vi "Launcher - gRPC Client.vi"(6 "Worker Alias":string="gRPC Client", 8 "error in":errorcluster, 9 "Initialization Data":T1, 11 "gRPC Client in":refnum<class "gRPC Client.lvclass">) -> (0 "error out":errorcluster)   [LabVIEW 2023]
doc: "This VI launches the Head Worker of a Workers application."
uses:
  Workers/gRPC Client/Initialization Data.ctl
  Workers/gRPC Client/Response Cases.ctl
  <vilib>/gRPC/LabVIEW gRPC Library/Shared/grpcId.ctl
  Workers/gRPC Client/gRPC Client.lvclass
  C:/Program Files (x86)/National Instruments/LabVIEW 2023/vi.lib/addons/_Workers/Library/Classes/Worker/Worker.lvclass
  <vilib>/addons/_Workers/Debugger/Debug Client/Debug Client.lvlib
  <vilib>/gRPC/LabVIEW gRPC Library/grpc-lvsupport-release.lvlib
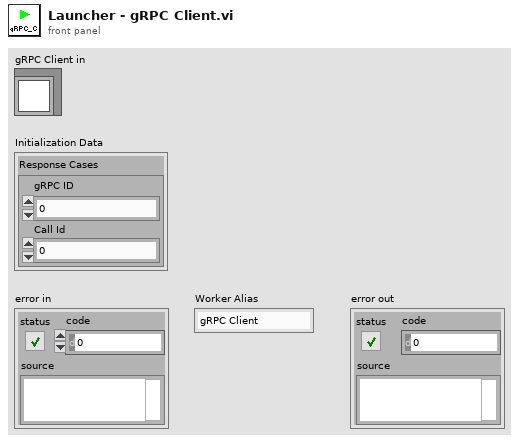
[diagram p1: front panel]
types:
  T1 = typedef "gRPC Client.lvclass/Initialization Data.ctl" = cluster{"Response Cases":T2}
  T2 = typedef "gRPC Client.lvclass/Response Cases.ctl" = cluster{"gRPC ID":T3, "Call Id":T3}
  T3 = typedef "grpc-lvsupport-release.lvlib/grpcId.ctl" = u64
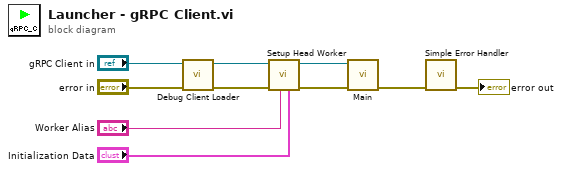
[diagram p0: block diagram]
diagram:
  n1 = call <vilib>:"Debug Client Loader.vi"("error in (no error)"="error in", "Worker_"="gRPC Client in") -> ("error out"=w3:errorcluster, "Worker_out"=w1:refnum<class "gRPC Client.lvclass">)  [unwired: 8 in]
  n2 = call-dynamic "Setup Head Worker.vi"("Initalization Data"="Initialization Data", "Worker Alias"="Worker Alias", "error in"=w3, "Worker_"=w1) -> ("error out"=w10:errorcluster, "Worker_out"=w7:refnum<class "gRPC Client.lvclass">)  [unwired: 6 in]
  n3 = call-dynamic "Main.vi"("error in"=w10, "gRPC Client in"=w7) -> ("error out"=w8:errorcluster)  [unwired: 8 in, 1 out]
  n4 = call <vilib>:"Simple Error Handler.vi"("error in (no error)"=w8) -> ("error out"=→"error out":errorcluster)  [unwired: 4 in, 4 out]
